vi "CRYTest IOName Array.vi"(10 "Name In":string[][](array[string]), 11 "Channel Info In":T1[](array[typedef]) {"Coupling" items=["Default"=-1, "RSE"=10083, "NRSE"=10078, "Differential"=10106, "Pseudodifferential"=12529]; "term config" items=["Default"=-1, "RSE"=10083, "NRSE"=10078, "Differential"=10106, "Pseudodifferential"=12529]; "Anti-aliasing Factor (%fs)" format="%.2f"}) -> (1 "Duplication Flag":bool, 2 "Name Out":string[][](array[string]), 3 "Channel Info Out":T1[](array[typedef]) {"Coupling" items=["Default"=-1, "RSE"=10083, "NRSE"=10078, "Differential"=10106, "Pseudodifferential"=12529]; "term config" items=["Default"=-1, "RSE"=10083, "NRSE"=10078, "Differential"=10106, "Pseudodifferential"=12529]; "Anti-aliasing Factor (%fs)" format="%.2f"})   [LabVIEW 2013]
uses:
  Typedef Control/CRYHardware Channel Info.ctl
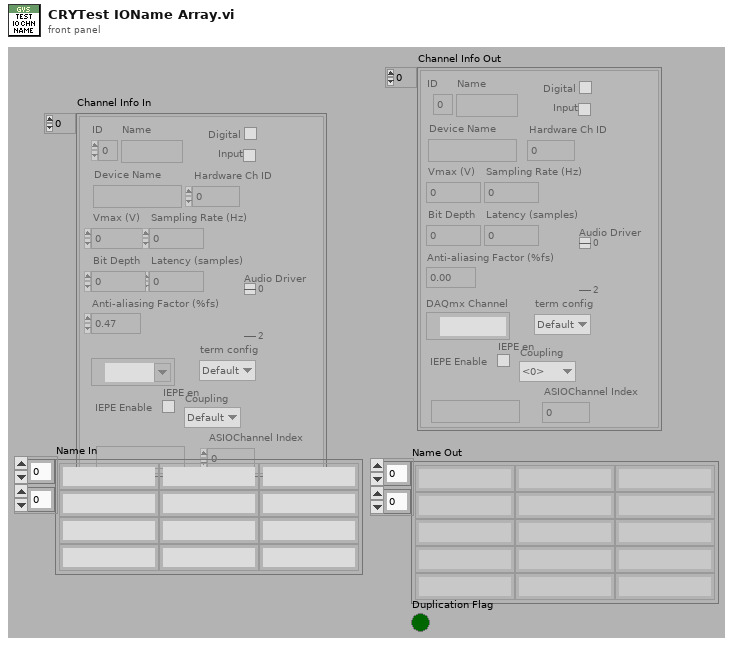
[diagram p1: front panel]
types:
  T1 = typedef "CRYHardware Channel Info.ctl" = cluster{"ID":i32, "Name":string, "Digital":bool, "Input":bool, "Device Name":string, "Hardware Ch ID":u8, "Vmax (V)":dbl, "Latency (samples)":dbl, "Sampling Rate (Hz)":u32, "Bit Depth":u32, "Anti-aliasing Factor (%fs)":sgl, "DAQmx Channel":tag, "term config":i32, "Coupling":i32, "IEPE en":bool, "ASIOChannel Name":string, "Audio Driver":u16, "ASIOChannel Index":u8}
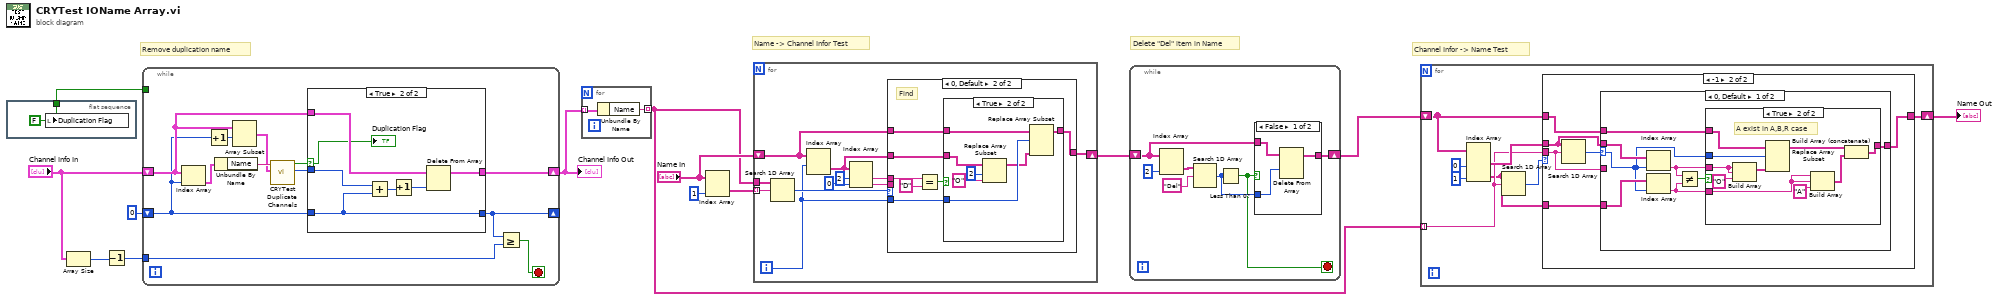
[diagram p0: block diagram]
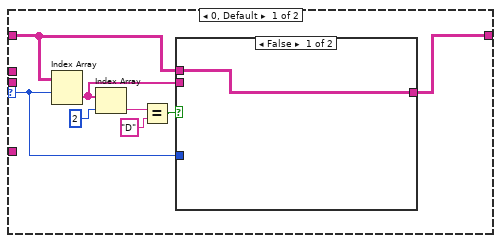
[diagram p2: hidden frame]
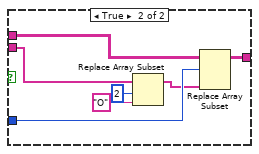
[diagram p3: hidden frame]
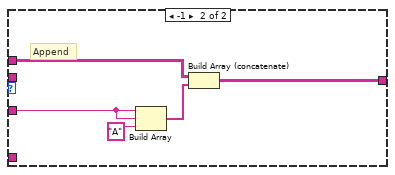
[diagram p5: hidden frame]
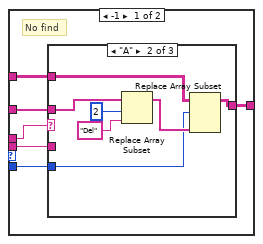
[diagram p7: hidden frame]
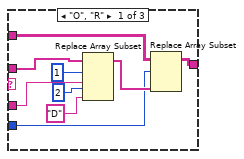
[diagram p8: hidden frame]
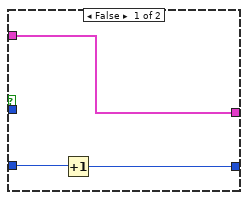
[diagram p11: hidden frame]
diagram:
  # "Channel Infor -> Name Test"
  # "Delete \"Del\" item in Name"
  # "Name -> Channel Infor Test"
  # "Remove duplication name"
  n1 = flat-sequence {
    tunnel: [w14] -> w9
    frame #0 {
      w14 = FALSE ("Exist Flag")
      n2 = local write "Duplication Flag"(w14) -> ()
    }
  }
  n3 = Array Size(array="Channel Info In") -> (size(s)=w11:i32)
  n4 = Decrement(x=w11) -> (x-1=w10:i32)
  n5 = while {
    tunnel: w10 -> [w22]
    shift-right: [w23] -> _
    shift-left: 0 -> [w18]
    shift-right: [w20] -> w4
    shift-left: "Channel Info In" -> [w19]
    tunnel: w9 -> [_]
    stop <- w21 stop-if-true
    n6 = Index Array(array=w19, index=w18) -> (element=w15:T1)
    n7 = Increment(x=w18) -> (x+1=w17:i32)
    n8 = Unbundle By Name(w15) -> ("Name"=w26:string)
    n9 = Array Subset(array=w19, index=w17) -> (w16:T1[])  [unwired: 1 in]
    n10 = call "CRYTest Duplicate Channels.vi"("Channel Info"=w16, "Channel Name"=w26) -> ("index of element"=w24:i32, "Exist Flag"=w25:bool)  [unwired: 8 in]
    n11 = case shown="True" w25 {
      selector: w25 -> [_ w30]
      tunnel: w24 -> [_ w33]
      tunnel: w18 -> [w29 w34]
      tunnel: [w28 w34] -> w23
      tunnel: w19 -> [w27 w36]
      tunnel: [w27 w35] -> w20
      frame False {
        n12 = Increment(x=w29) -> (x+1=w28:i32)
      }
      frame True {
        n13 = Add(x=w33, y=w34) -> (x+y=w32:i32)
        n14 = Increment(x=w32) -> (x+1=w31:i32)
        n15 = Delete From Array(array=w36, index=w31) -> (array with subset deleted=w35:T1[])  [unwired: 1 in, 1 out]
        "Duplication Flag" <- w30
      }
    }
    n16 = Greater Or Equal?(x=w23, y=w22) -> (x >= y?=w21:bool)
  }
  "Channel Info Out" <- w4
  n17 = for {
    tunnel: w4 -> [w38] mode=indexing
    tunnel: [w37] -> w2 mode=indexing
    n18 = Unbundle By Name(w38) -> ("Name"=w37:string)
  }
  n19 = Index Array(array="Name In", index (col)=1 ("disabled index (col)")) -> (element=w7:string[])  [unwired: 1 in]
  n20 = for {
    tunnel: w7 -> [w49] mode=indexing
    shift-right: [w41] -> w5
    shift-left: "Name In" -> [w43]
    tunnel: w2 -> [w48]
    i -> [w42]
    n21 = Search 1D Array(1D array=w48, element=w49) -> (index of element=w46:i32)  [unwired: 1 out]
    n22 = Index Array(array=w43, index (row)=w42) -> (element=w45:string[])  [unwired: 1 in]
    n23 = Index Array(array=w45, index #1=2 ("index"), index #2=0 ("index")) -> (element #1=w44:string, element #2=w39:string)
    n24 = case shown="0, Default" w46 {
      tunnel: w45 -> [w53 w76]
      tunnel: w44 -> [w55 w79]
      tunnel: w43 -> [w54 w75]
      tunnel: w42 -> [w52 w74]
      tunnel: [w51 w73] -> w41
      tunnel: w39 -> [w50 _]
      frame -1 {
        # "No find"
        n25 = case shown="\"A\"" w55 {
          tunnel: w54 -> [w62 w69 w72]
          tunnel: w53 -> [w64 w71 _]
          tunnel: w52 -> [w61 w68 _]
          tunnel: [w60 w67 w72] -> w51
          tunnel: w50 -> [w57 _ _]
          frame "O", "R" {
            n26 = Replace Array Subset(array=w64, new element #1=w57, index #1=1 ("index"), new element #2="D" ("new element/subarray"), index #2=2 ("index")) -> (w63:string[])
            n27 = Replace Array Subset(array=w62, new element=w63, index (row)=w61) -> (w60:string[][])  [unwired: 1 in]
          }
          frame "A" {
            n28 = Replace Array Subset(array=w71, new element="Del" ("new element/subarray"), index=2) -> (w70:string[])
            n29 = Replace Array Subset(array=w69, new element=w70, index (row)=w68) -> (w67:string[][])  [unwired: 1 in]
          }
          frame Default {
          }
        }
      }
      frame 0, Default {
        # "Find"
        n30 = Equal?(x=w79, y="D") -> (x = y?=w77:bool)
        n31 = case shown="True" w77 {
          tunnel: w76 -> [_ w85]
          tunnel: w75 -> [w80 w84]
          tunnel: w74 -> [_ w83]
          tunnel: [w80 w81] -> w73
          frame False {
          }
          frame True {
            n32 = Replace Array Subset(array=w85, new element="O" ("new element/subarray"), index=2) -> (w82:string[])
            n33 = Replace Array Subset(array=w84, new element=w82, index (row)=w83) -> (w81:string[][])  [unwired: 1 in]
          }
        }
      }
    }
  }
  n34 = while {
    shift-right: [w90] -> w3
    shift-left: w5 -> [w91]
    stop <- w88 stop-if-true
    n35 = Index Array(array=w91, index (col)=2 ("disabled index (col)")) -> (element=w93:string[])  [unwired: 1 in]
    n36 = Search 1D Array(1D array=w93, element="Del") -> (index of element=w89:i32)  [unwired: 1 out]
    n37 = Less Than 0?(x=w89) -> (x < 0?=w88:bool)
    n38 = case shown="False" w88 {
      tunnel: w91 -> [w97 w98]
      tunnel: [w95 w98] -> w90
      tunnel: w89 -> [w96 _]
      frame False {
        n39 = Delete From Array(array=w97, index (row)=w96) -> (array with subset deleted=w95:string[][])  [unwired: 2 in, 1 out]
      }
      frame True {
      }
    }
  }
  n40 = for {
    shift-right: [w100] -> w1
    shift-left: w3 -> [w101]
    tunnel: w2 -> [w103] mode=indexing
    n41 = Index Array(array=w101, index (col) #1=0 ("disabled index (col)"), index (col) #2=1 ("index (col)")) -> (element #1=w104:string[], element #2=w99:string[])  [unwired: 2 in]
    n42 = Search 1D Array(1D array=w99, element=w103) -> (index of element=w102:i32)  [unwired: 1 out]
    n43 = case shown="-1" w102 {
      selector: w102 -> [w108 _]
      tunnel: w104 -> [_ w124]
      tunnel: w103 -> [_ w125]
      tunnel: w101 -> [w111 w127]
      tunnel: [w110 w126] -> w100
      tunnel: w99 -> [_ w123]
      frame 0, Default {
        n44 = Index Array(array=w111, index (row)=w108) -> (element=w107:string[])  [unwired: 1 in]
        n45 = Index Array(array=w107, index=2 ("disabled index (col)")) -> (element=w113:string)
        n46 = Equal?(x=w113, y="D") -> (x = y?=w109:bool)
        n47 = case shown="False" w109 {
          tunnel: w111 -> [w115 w122]
          tunnel: [w115 w121] -> w110
          tunnel: w108 -> [_ w120]
          tunnel: w107 -> [_ w117]
          frame False {
          }
          frame True {
            n48 = Replace Array Subset(array=w117, new element="O" ("new element/subarray"), index=2) -> (w116:string[])
            n49 = Replace Array Subset(array=w122, new element=w116, index (row)=w120) -> (w121:string[][])  [unwired: 1 in]
          }
        }
      }
      frame -1 {
        n50 = Search 1D Array(1D array=w124, element=w125) -> (index of element=w128:i32)  [unwired: 1 out]
        n51 = case shown="0, Default" w128 {
          selector: w128 -> [w130 _]
          tunnel: w127 -> [w133 w152]
          tunnel: [w134 w151] -> w126
          tunnel: w125 -> [_ w150]
          tunnel: w124 -> [w136 _]
          tunnel: w123 -> [w135 _]
          frame 0, Default {
            n52 = Index Array(array=w136, index=w130) -> (element=w131:string)
            n53 = Index Array(array=w135, index=w130) -> (element=w132:string)
            n54 = Not Equal?(x=w131, y=w132) -> (x != y?=w129:bool)
            n55 = case shown="True" w129 {
              tunnel: [w137 w144] -> w134
              tunnel: w133 -> [w137 w143]
              tunnel: w132 -> [_ w142]
              tunnel: w131 -> [_ w141]
              tunnel: w130 -> [_ w138]
              frame False {
                # "no this case"
              }
              frame True {
                # "A exist in A,B,R case"
                n56 = Build Array(w141, w141, "O" ("Name")) -> (w139:string[])
                n57 = Replace Array Subset(array=w143, new element=w139, index (row)=w138) -> (w145:string[][])  [unwired: 1 in]
                n58 = Build Array(w142, w142, "A" ("Name")) -> (w146:string[])
                n59 = Build Array (concatenate)(w145, w146) -> (w144:string[][])
              }
            }
          }
          frame -1 {
            # "Append"
            n60 = Build Array(w150, w150, "A" ("Name")) -> (w148:string[])
            n61 = Build Array (concatenate)(w152, w148) -> (w151:string[][])
          }
        }
      }
    }
  }
  "Name Out" <- w1
